vi "Tektronix 7000 Series Read Waveform from File Interactive.vi"() -> ()   [LabVIEW 2015]
doc: "This example VI illustrates how to read data from a file.\nTo analyze an area of interest in detail, use the cursor to select the starting and ending positions. This VI then reads the file again and acquires more data points between the starting and ending positions."
uses:
  <instrlib>/Tektronix 7000 Series/Tektronix 7000 Series.lvlib
panel:
  in  "Waveform Graph":waveform(sgl)(graph)={"t0"=timestamp(0.0019774760585278273 s since 1904-01-01), "dt"=4.999999987376214e-07, "Y"=[]}
  in  "Path":path=path "C:/data.txt"
  in  "stop 2":bool
  # "(c) 2006 - 2016 National Instruments Corporation.  ALL RIGHTS RESERVED."
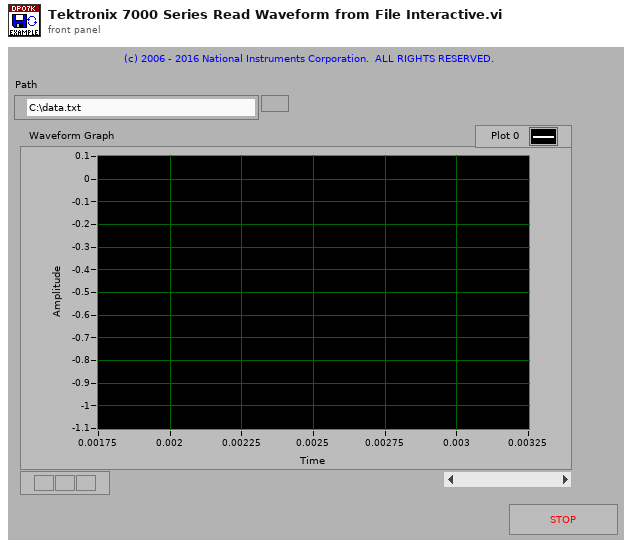
[diagram p1: front panel]
types:
  T1 = cluster{"t0":timestamp, "det x":sgl, "data":sgl[]}
  T2 = enum16{"open", "open or create", "create or replace", "create", "open (read only)"}
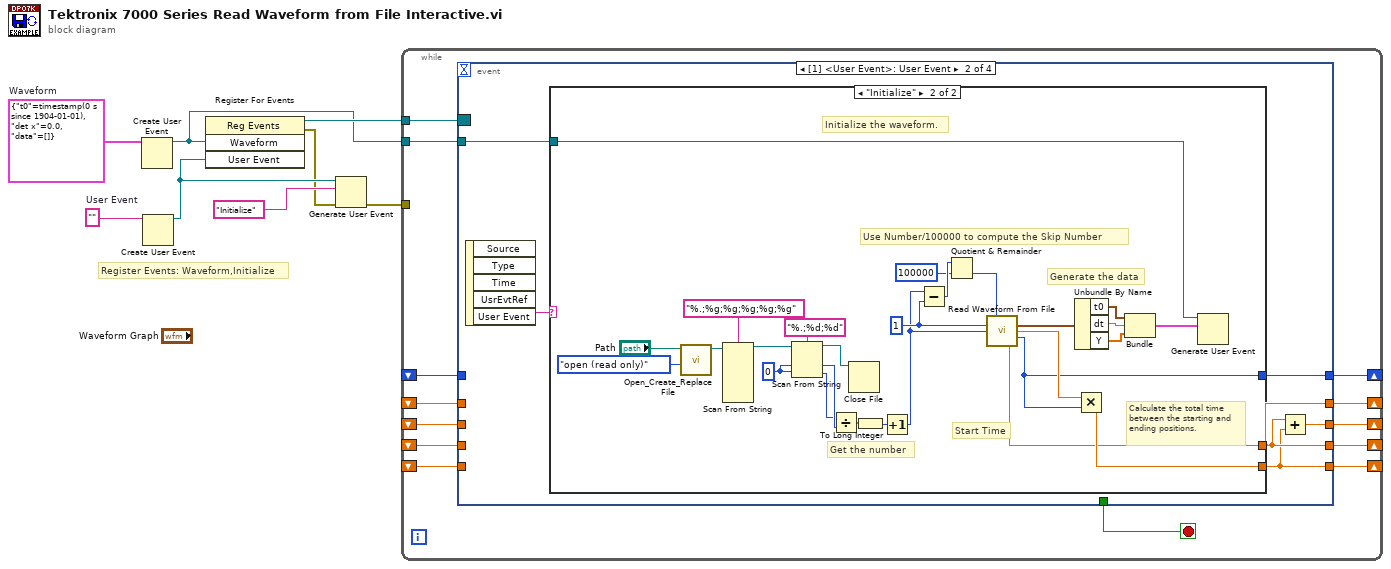
[diagram p0: block diagram]
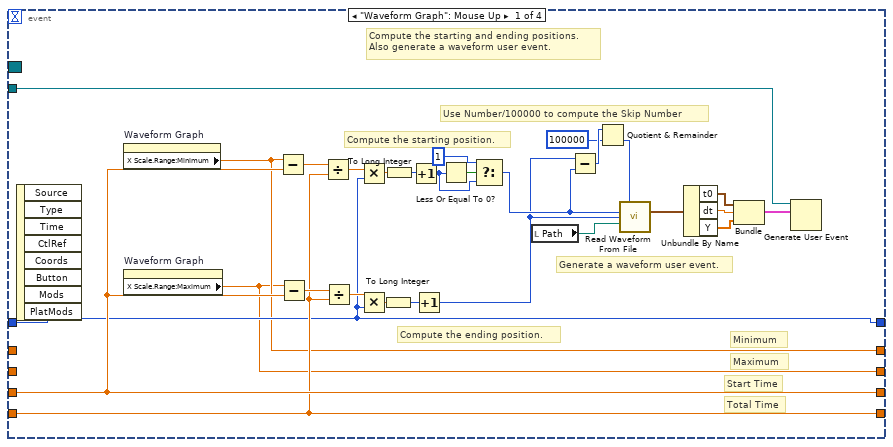
[diagram p2: hidden frame]
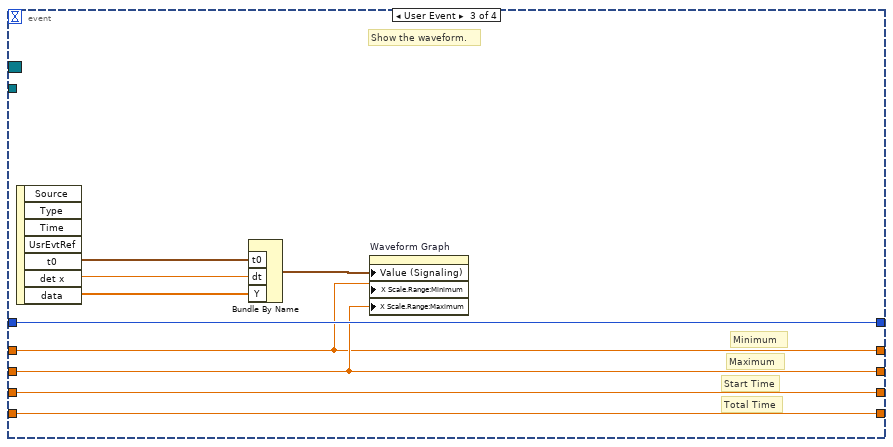
[diagram p4: hidden frame]
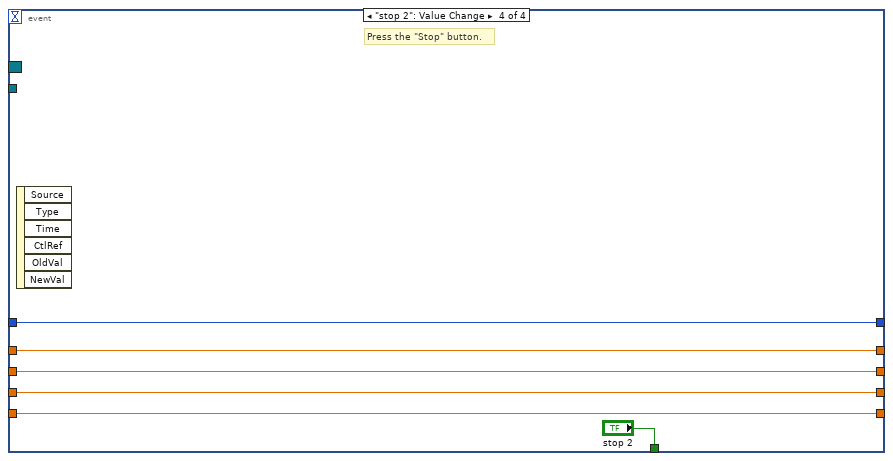
[diagram p5: hidden frame]
diagram:
  w1 = T1 {"t0"=timestamp(0 s since 1904-01-01), "det x"=0.0, "data"=[]}  # Waveform
  w7 = ""  # User Event
  # "Register Events: Waveform,Initialize"
  n1 = Create User Event(user event datatype=w1) -> (user event=w3:refnum<user-event>)  [unwired: 1 in, 1 out]
  n2 = Create User Event(user event datatype=w7) -> (user event=w6:refnum<user-event>)  [unwired: 1 in, 1 out]
  n3 = register-events(w3, w6) -> (reference out=w8:refnum<event-registration>, error out=w4:errorcluster)  [unwired: 2 in]
  n4 = Generate User Event(user event=w6, event data cluster="Initialize" ("event data"), error in=w4) -> (error out=w2:errorcluster)  [unwired: 1 in, 1 out]
  n5 = while {
    tunnel: w8 -> [w21]
    tunnel: w3 -> [w20]
    shift-right: [w19] -> _
    shift-left: _ -> [w16]
    shift-right: [w18] -> _
    shift-left: _ -> [w17]
    tunnel: w2 -> [_]
    shift-right: [w15] -> _
    shift-left: _ -> [w13]
    shift-right: [w14] -> _
    shift-left: _ -> [w12]
    shift-right: [w10] -> _
    shift-left: _ -> [w9]
    stop <- w11 stop-if-true
    n6 = event shown="[1] <User Event>: User Event" {
      selector: w21 -> [_ _ _ _]
      dyn-events: _ -> [_ _ _ _]
      timeout: _ -> [_ _ _ _]
      tunnel: w20 -> [w45 w54 _ _]
      tunnel: [w44 w52 w90 w95] -> w19
      tunnel: [w43 w51 w91 w94] -> w18
      tunnel: w16 -> [w44 _ w90 w95]
      tunnel: w17 -> [w43 _ w91 w94]
      tunnel: [w36 w52 w87 w97] -> w15
      tunnel: [w35 w53 w88 w96] -> w14
      tunnel: w13 -> [_ _ w87 w97]
      tunnel: w12 -> [_ _ w88 w96]
      tunnel: [_ _ _ "stop 2"] -> w11
      tunnel: [w41 w50 w89 w92] -> w10
      tunnel: w9 -> [w41 _ w89 w92]
      event "Waveform Graph": Mouse Up {
        # "Use Number/100000 to compute the Skip Number"
        # "Total Time"
        # "Start Time"
        # "Maximum"
        # "Minimum"
        # "Generate a waveform user event."
        # "Compute the ending position."
        # "Compute the starting position."
        # "Compute the starting and ending positions.\nAlso generate a waveform user event."
        n7 = event-data() -> ()  [unwired: 1 in, 8 out]
        n8 = property on="Waveform Graph" class="WFGraph (strict)"() -> ("X Scale.Range:Minimum"=w36:dbl)  [unwired: 2 in, 2 out]
        n9 = property on="Waveform Graph" class="WFGraph (strict)"() -> ("X Scale.Range:Maximum"=w35:dbl)  [unwired: 2 in, 2 out]
        n10 = Subtract(x=w36, y=w44) -> (x-y=w49:dbl)
        n11 = Subtract(x=w35, y=w44) -> (x-y=w48:dbl)
        n12 = Divide(x=w49, y=w43) -> (x/y=w47:dbl)
        n13 = Divide(x=w48, y=w43) -> (x/y=w46:dbl)
        n14 = Multiply(x=w47, y=w41) -> (x*y=w29:dbl)
        n15 = Multiply(x=w46, y=w41) -> (x*y=w37:dbl)
        n16 = To Long Integer(number=w37) -> (32bit integer=w27:i32)
        n17 = To Long Integer(number=w29) -> (32bit integer=w28:i32)
        n18 = Increment(x=w28) -> (x+1=w24:i32)
        n19 = Increment(x=w27) -> (x+1=w22:i32)
        n20 = Less Or Equal To 0?(x=w24) -> (x <= 0?=w26:bool)
        n21 = Select(t=i16 1, s=w26, f=w24) -> (s? t:f=w23:i32)
        n22 = local read "Path"() -> (w42:path)
        n23 = Subtract(x=w22, y=w23) -> (x-y=w40:i32)
        n24 = Quotient & Remainder(x=w40, y=100000) -> (floor(x/y)=w38:i32)  [unwired: 1 out]
        n25 = call <instrlib>:"Read Waveform From File.vi"("Skip N Points (1)"=w38, "Start Point (1)"=w23, "End Point (10000)"=w22, "Filename (C:\\data.txt)"=w42) -> ("Waveform Graph"=w31:waveform(sgl))  [unwired: 6 in, 5 out]
        n26 = Unbundle By Name(w31) -> ("t0"=w34:timestamp, "dt"=w33:dbl, "Y"=w32:sgl[])
        n27 = Bundle("t0"=w34, "dt"=w33, "Y"=w32) -> (w30:cluster{"t0":timestamp, "dt":dbl, "Y":sgl[]})  [unwired: 1 in]
        n28 = Generate User Event(user event=w45, event data cluster=w30) -> ()  [unwired: 2 in, 2 out]
      }
      event User Event {
        n29 = event-data() -> ("User Event"=w55:string)  [unwired: 1 in, 4 out]
        n30 = case shown="\"Initialize\"" w55 {
          tunnel: w54 -> [_ w82]
          tunnel: [_ w80] -> w52
          tunnel: [_ w81] -> w51
          tunnel: [_ w78] -> w50
          frame "False", Default {
          }
          frame "Initialize" {
            w66 = 0 ("default value 6")
            w71 = 1 ("Start Point (1)")
            # "Generate the data"
            # "Get the number"
            # "Use Number/100000 to compute the Skip Number"
            # "Initialize the waveform."
            # "Start Time"
            # "Calculate the total time between the starting and ending positions."
            n31 = call <vilib>:"Open_Create_Replace File.vi"("function (open:0)"=T2."open (read only)", "file path"="Path") -> ("refnum"=w72:refnum<file>)  [unwired: 6 in, 3 out]
            n32 = Scan From String("%.;%g;%g;%g;%g;%g" ("format string"), w72) -> (w68:refnum<file>)  [unwired: 11 in, 1 out]
            n33 = Scan From String("%.;%d;%d" ("format string"), w68, default 1=w66, default 2=w66) -> (w67:refnum<file>, output 1=w65:i32, output 2=w64:i32)  [unwired: 1 in, 1 out]
            n34 = Divide(x=w64, y=w65) -> (x/y=w63:dbl)
            n35 = Close File(refnum=w67) -> ()  [unwired: 1 in, 2 out]
            n36 = To Long Integer(number=w63) -> (32bit integer=w61:i32)
            n37 = Increment(x=w61) -> (x+1=w62:i32)
            n38 = Subtract(x=w62, y=w71) -> (x-y=w77:i32)
            n39 = Quotient & Remainder(x=w77, y=100000) -> (floor(x/y)=w70:i32)  [unwired: 1 out]
            n40 = call <instrlib>:"Read Waveform From File.vi"("Skip N Points (1)"=w70, "Start Point (1)"=w71, "End Point (10000)"=w62) -> ("Waveform Graph"=w60:waveform(sgl), "Time Interval"=w79:sgl, "Count"=w78:i32, "Start Time"=w80:sgl)  [unwired: 7 in, 2 out]
            n41 = Unbundle By Name(w60) -> ("t0"=w59:timestamp, "dt"=w58:dbl, "Y"=w57:sgl[])
            n42 = Multiply(x=w79, y=w78) -> (x*y=w81:sgl)
            n43 = Bundle("t0"=w59, "dt"=w58, "Y"=w57) -> (w56:cluster{"t0":timestamp, "dt":dbl, "Y":sgl[]})  [unwired: 1 in]
            n44 = Generate User Event(user event=w82, event data cluster=w56) -> ()  [unwired: 2 in, 2 out]
          }
        }
        n45 = Add(x=w52, y=w51) -> (x+y=w53:sgl)
      }
      event User Event {
        # "Total Time"
        # "Start Time"
        # "Maximum"
        # "Minimum"
        # "Show the waveform."
        n46 = event-data() -> ("t0"=w83:timestamp, "det x"=w85:sgl, "data"=w84:sgl[])  [unwired: 1 in, 4 out]
        n47 = Bundle By Name ("Build Waveform")("t0"=w83, "dt"=w85, "Y"=w84) -> (w86:waveform(sgl))  [unwired: 1 in]
        n48 = property on="Waveform Graph" class="WFGraph (strict)"("Value (Signaling)"=w86, "X Scale.Range:Minimum"=w87, "X Scale.Range:Maximum"=w88) -> ()  [unwired: 2 in, 2 out]
      }
      event "stop 2": Value Change {
        # "Press the \"Stop\" button."
        n49 = event-data() -> ()  [unwired: 1 in, 6 out]
      }
    }
  }
